vi "Obtain-settings-file-paths.vi"(8 "error in":errorcluster, 11 "Data ref. in":refnum<data-value>) -> (0 "error IO":errorcluster, 1 "Path ok?":bool, 2 "File paths":path[](array[path]), 3 "Data ref.":refnum<data-value>)   [LabVIEW 2013, in "CameraVision.lvlib" / "CV-Main.lvclass"]
doc: "This function determines whether the save is programmatically started (start of acquisition) or not, by checking the enabled state of the 'Start' button. Enabled means a user initiated save.\n\nIn case of an automated save the returned file paths are that of the user-selected storage directory with the base file name, appended with the file extension (.xml) and that of the directory and default name of the last-used-settings file (<Application>\\Program data\\last.xml).\n\nIn the case of a user save a dialog is displayed to ask the user to choose a filepath and name.\n\nWhen a file with the same path and name already exists, a warning message is displayed which allows the user to cancel or confirm the save operation."
uses:
  CV-Main.lvclass
  UI/Popup-messages.ctl
  CV-Main.lvclass/CV-Main.ctl
  Storage/CV-Storage.lvclass/CV-Storage.ctl
  Storage/Read Storage directory.vi
  Storage/Read Base file name.vi
  Storage/Read Base path.vi
  Read Storage params.vi
  Storage/CV-Storage.lvclass
  UI/CV-UI.lvclass
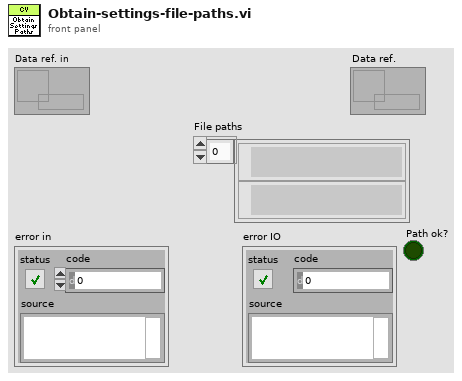
[diagram p1: front panel]
types:
  T1 = typedef "CameraVision.lvlib/CV-UI.lvclass/Popup-messages.ctl" = enum16{"Error-Black image", "Error-Camera config file", "Error-Camera connect", "Error-Grabber init", "Error-Camera setting", "Error-Image offset", "Error-Image import", "Error-Settings file not exist", "Error-Timing source", "Conflict-Filters", "Conflict-Map", "Conflict-Framerate", "Conflict-Charact", "Conflict-Temperature field", "Conflict-Temperature value", "Conflict-Storage-Binary image", "Conflict-Storage-Corrected image", "Conflict-Storage-Map", "Conflict-Storage-Charact", "Conflict-Storage-Temperature field", "Conflict-Storage-Temperature value", "Warning-File exist", "Warning-Parameter reset", "Warning-User cancel", "Info-Images imported"}
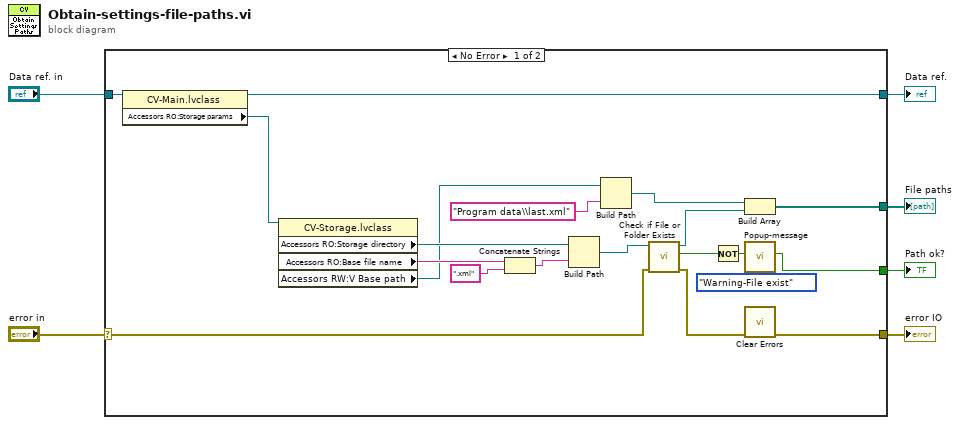
[diagram p0: block diagram]
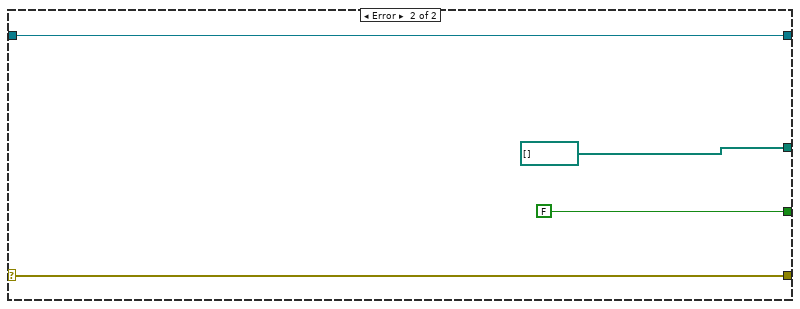
[diagram p2: hidden frame]
diagram:
  n1 = case shown="No Error" "error in" {
    selector: "error in" -> [w10 w30]
    tunnel: [w26 FALSE ("T button?")] -> w6
    tunnel: [w25 path[] []] -> w5
    tunnel: [w24 w30] -> w3
    tunnel: "Data ref. in" -> [w21 w28]
    tunnel: [w11 w28] -> w1
    frame No Error {
      n2 = property class="CV-Main.lvclass"(reference=w21) -> (reference out=w11:refnum<data-value>, "Accessors RO:Storage params"=w20:refnum<data-value>)  [unwired: 1 in, 1 out]
      n3 = property class="CV-Storage.lvclass"(reference=w20) -> ("Accessors RO:Storage directory"=w22:path, "Accessors RO:Base file name"=w23:string, "Accessors RW:V Base path"=w19:path)  [unwired: 1 in, 2 out]
      n4 = Concatenate Strings(w23, ".xml" ("string")) -> (w17:string)
      n5 = Build Path(base path=w22, name or relative path=w17) -> (appended path=w14:path)
      n6 = Build Path(base path=w19, name or relative path="Program data\\last.xml" ("string")) -> (appended path=w12:path)
      n7 = call <vilib>:"Check if File or Folder Exists.vi"("error in (no error)"=w10, "path"=w14) -> ("error out"=w9:errorcluster, "file or folder exists?"=w16:bool, "dup path"=w13:path)  [unwired: 7 in]
      n8 = Not(x=w16) -> (.not. x?=w7:bool)
      n9 = Build Array(w12, w13) -> (w25:path[])
      n10 = call "Popup-message.vi"("Message"=Popup-messages."Warning-File exist", "Ignore?"=w7) -> ("Return"=w26:bool)  [unwired: 9 in]
      n11 = call <vilib>:"Clear Errors.vi"("error in (no error)"=w9) -> ("error out"=w24:errorcluster)  [unwired: 6 in]
    }
    frame Error {
    }
  }
  "Path ok?" <- w6
  "File paths" <- w5
  "error IO" <- w3
  "Data ref." <- w1
